vi "Get Pot Zero.vi"() -> (2 "Left Pot 0":dbl, 3 "Right Pot 0":dbl)   [LabVIEW 2015]
uses:
  Common Code/Dashboard Communication/Dashboard Control Data.ctl
  Common Code/Shooter Presets.ctl
  Common Code/Shot Presets.ctl
  Common Code/Encoder Control.ctl
  Common Code/Drivetrain Settings.ctl
  Common Code/Goal Vision Packet.ctl
  Common Code/Dashboard Drivetrain Command.ctl
  Common Code/Drivetrain Vision.ctl
  Common Code/Intake Command Cluster.ctl
  Common Code/Ball Tracking Command Cluster.ctl
  Common Code/Ball Vision Packet.ctl
  Common Code/Tracking Mode.ctl
  Robot Global Data.vi
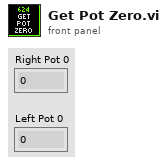
[diagram p1: front panel]
types:
  T1 = typedef "Dashboard Control Data.ctl" = cluster{"Shooter Presets":T2, "Encoder Control":T4, "Steer PID output":cluster{"output high":dbl, "output low":dbl}, " Steer PID gains":cluster{"proportional gain (Kc)":dbl, "integral time (Ti, min)":dbl, "derivative time (Td, min)":dbl}, "Drivetrain Settings":T5, "Vision Packet":T6, "Dashboard Drivetrain Command":T7, "Intake Command Cluster":T9, "Info/Command Cluster":T10, "Ball Vision Packet":T11}
  T2 = typedef "Shooter Presets.ctl" = cluster{"Batter Shot":T3, "Low Bar Curve Shot":T3, "Deep Middle Shot":T3, "Manual Shot":T3, "Left Ticks Per Rotation":dbl, "Right Ticks Per Rotation":dbl, "Low Bar Shot":T3, "Shooter RPM Tolerance":dbl, "IIR Filter Power":dbl, "Trigger Power":dbl, "Fire from Load Delay":i32, "Angle Pot Scale Factor":dbl, "Angle Pot Zero":dbl, "Shooter Deck Length":dbl, "String Pot Dist From Pivot":dbl, "Angle PID gains":cluster{"proportional gain (Kc)":dbl, "integral time (Ti, min)":dbl, "derivative time (Td, min)":dbl}, "Angle Motor Output Range":cluster{"output high":dbl, "output low":dbl}, "Shooter Angle Tolerance":dbl, "Vision Shoot m":dbl, "Vision Shoot b":dbl, "Dist from Axis Cam to Pivot":dbl, "High Goal Center Height":dbl}
  T3 = typedef "Shot Presets.ctl" = cluster{"Left Wheel RPM":dbl, "Right Wheel RPM":dbl, "Angle":dbl}
  T4 = typedef "Encoder Control.ctl" = cluster{"Right Tick Constant":dbl, "Left Tick Constant":dbl, "Reset?":bool, "Y Dist":cluster{"PID gains":cluster{"proportional gain (Kc)":dbl, "integral time (Ti, min)":dbl, "derivative time (Td, min)":dbl}}, "Y Stop Thresh":dbl, "Y Stop Speed":dbl}
  T5 = typedef "Drivetrain Settings.ctl" = cluster{"Gyro Tolerance":dbl, "Throttle Ramp (ms)":dbl, "Angular rate compensation":bool, "Throttle to Rate Scale":dbl, "Rate compensation gain":dbl}
  T6 = typedef "Goal Vision Packet.ctl" = cluster{"Distance":dbl, "Center X":dbl, "Center Y":dbl, "Found Target?":bool}
  T7 = typedef "Dashboard Drivetrain Command.ctl" = cluster{"Drivetrain Vision":T8, "Vision Scale Down Speed":dbl, "Vision PID gains":cluster{"proportional gain (Kc)":dbl, "integral time (Ti, min)":dbl, "derivative time (Td, min)":dbl}}
  T8 = typedef "Drivetrain Vision.ctl" = cluster{"High parameters":dbl, "Low parameters":dbl}
  T9 = typedef "Intake Command Cluster.ctl" = cluster{"Suck Speed":dbl, "Spit Speed":dbl, "Right Pot 0":dbl, "Left Pot 0":dbl, "Trigger Power":dbl, "Raise Speed":dbl, "Lower Speed":dbl}
  T10 = typedef "Ball Tracking Command Cluster.ctl" = cluster{"Distance to Ball":dbl, "Desired Angle":dbl, "Command":enum16{"Turn to Ball", "Turn to Angle", "Get Distance"}, "Pixels from Center":dbl}
  T11 = typedef "Ball Vision Packet.ctl" = cluster{"Ball Detected?":bool, "Distance to Ball":dbl, "Desired Angle":dbl, "Pixels from Center":dbl, "Tracking mode":T12}
  T12 = typedef "Tracking Mode.ctl" = enum16{"Turn to Ball", "Turn to Angle"}
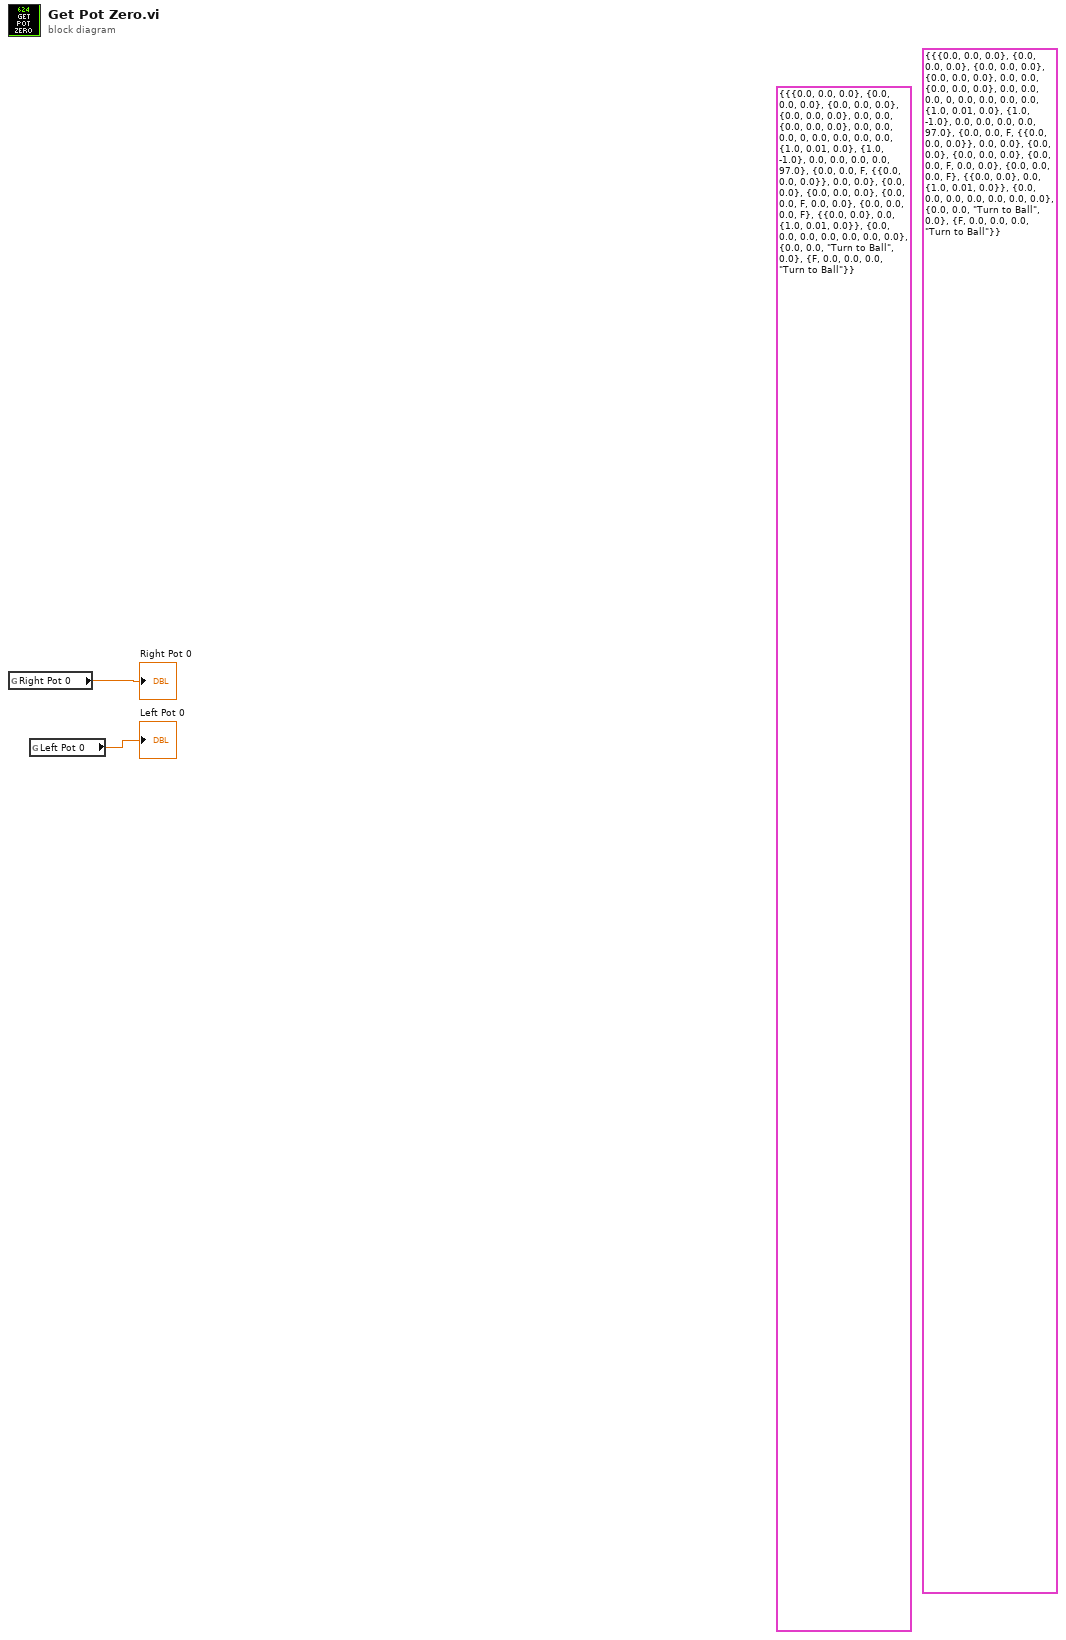
[diagram p0: block diagram]
diagram:
  (unwired) T1 {"Shooter Presets"={"Batter Shot"={"Left Wheel RPM"=0.0, "Right Wheel RPM"=0.0, "Angle"=0.0}, "Low Bar Curve Shot"={"Left Wheel RPM"=0.0, "Right Wheel RPM"=0.0, "Angle"=0.0}, "Deep Middle Shot"={"Left Wheel RPM"=0.0, "Right Wheel RPM"=0.0, "Angle"=0.0}, "Manual Shot"={"Left Wheel RPM"=0.0, "Right Wheel RPM"=0.0, "Angle"=0.0}, "Left Ticks Per Rotation"=0.0, "Right Ticks Per Rotation"=0.0, "Low Bar Shot"={"Left Wheel RPM"=0.0, "Right Wheel RPM"=0.0, "Angle"=0.0}, "Shooter RPM Tolerance"=0.0, "IIR Filter Power"=0.0, "Trigger Power"=0.0, "Fire from Load Delay"=0, "Angle Pot Scale Factor"=0.0, "Angle Pot Zero"=0.0, "Shooter Deck Length"=0.0, "String Pot Dist From Pivot"=0.0, "Angle PID gains"={"proportional gain (Kc)"=1.0, "integral time (Ti, min)"=0.01, "derivative time (Td, min)"=0.0}, "Angle Motor Output Range"={"output high"=1.0, "output low"=-1.0}, "Shooter Angle Tolerance"=0.0, "Vision Shoot m"=0.0, "Vision Shoot b"=0.0, "Dist from Axis Cam to Pivot"=0.0, "High Goal Center Height"=97.0}, "Encoder Control"={"Right Tick Constant"=0.0, "Left Tick Constant"=0.0, "Reset?"=FALSE, "Y Dist"={"PID gains"={"proportional gain (Kc)"=0.0, "integral time (Ti, min)"=0.0, "derivative time (Td, min)"=0.0}}, "Y Stop Thresh"=0.0, "Y Stop Speed"=0.0}, "Steer PID output"={"output high"=0.0, "output low"=0.0}, " Steer PID gains"={"proportional gain (Kc)"=0.0, "integral time (Ti, min)"=0.0, "derivative time (Td, min)"=0.0}, "Drivetrain Settings"={"Gyro Tolerance"=0.0, "Throttle Ramp (ms)"=0.0, "Angular rate compensation"=FALSE, "Throttle to Rate Scale"=0.0, "Rate compensation gain"=0.0}, "Vision Packet"={"Distance"=0.0, "Center X"=0.0, "Center Y"=0.0, "Found Target?"=FALSE}, "Dashboard Drivetrain Command"={"Drivetrain Vision"={"High parameters"=0.0, "Low parameters"=0.0}, "Vision Scale Down Speed"=0.0, "Vision PID gains"={"proportional gain (Kc)"=1.0, "integral time (Ti, min)"=0.01, "derivative time (Td, min)"=0.0}}, "Intake Command Cluster"={"Suck Speed"=0.0, "Spit Speed"=0.0, "Right Pot 0"=0.0, "Left Pot 0"=0.0, "Trigger Power"=0.0, "Raise Speed"=0.0, "Lower Speed"=0.0}, "Info/Command Cluster"={"Distance to Ball"=0.0, "Desired Angle"=0.0, "Command"=enum."Turn to Ball", "Pixels from Center"=0.0}, "Ball Vision Packet"={"Ball Detected?"=FALSE, "Distance to Ball"=0.0, "Desired Angle"=0.0, "Pixels from Center"=0.0, "Tracking mode"=enum."Turn to Ball"}} ("Dashboard Control Data")
  (unwired) T1 {"Shooter Presets"={"Batter Shot"={"Left Wheel RPM"=0.0, "Right Wheel RPM"=0.0, "Angle"=0.0}, "Low Bar Curve Shot"={"Left Wheel RPM"=0.0, "Right Wheel RPM"=0.0, "Angle"=0.0}, "Deep Middle Shot"={"Left Wheel RPM"=0.0, "Right Wheel RPM"=0.0, "Angle"=0.0}, "Manual Shot"={"Left Wheel RPM"=0.0, "Right Wheel RPM"=0.0, "Angle"=0.0}, "Left Ticks Per Rotation"=0.0, "Right Ticks Per Rotation"=0.0, "Low Bar Shot"={"Left Wheel RPM"=0.0, "Right Wheel RPM"=0.0, "Angle"=0.0}, "Shooter RPM Tolerance"=0.0, "IIR Filter Power"=0.0, "Trigger Power"=0.0, "Fire from Load Delay"=0, "Angle Pot Scale Factor"=0.0, "Angle Pot Zero"=0.0, "Shooter Deck Length"=0.0, "String Pot Dist From Pivot"=0.0, "Angle PID gains"={"proportional gain (Kc)"=1.0, "integral time (Ti, min)"=0.01, "derivative time (Td, min)"=0.0}, "Angle Motor Output Range"={"output high"=1.0, "output low"=-1.0}, "Shooter Angle Tolerance"=0.0, "Vision Shoot m"=0.0, "Vision Shoot b"=0.0, "Dist from Axis Cam to Pivot"=0.0, "High Goal Center Height"=97.0}, "Encoder Control"={"Right Tick Constant"=0.0, "Left Tick Constant"=0.0, "Reset?"=FALSE, "Y Dist"={"PID gains"={"proportional gain (Kc)"=0.0, "integral time (Ti, min)"=0.0, "derivative time (Td, min)"=0.0}}, "Y Stop Thresh"=0.0, "Y Stop Speed"=0.0}, "Steer PID output"={"output high"=0.0, "output low"=0.0}, " Steer PID gains"={"proportional gain (Kc)"=0.0, "integral time (Ti, min)"=0.0, "derivative time (Td, min)"=0.0}, "Drivetrain Settings"={"Gyro Tolerance"=0.0, "Throttle Ramp (ms)"=0.0, "Angular rate compensation"=FALSE, "Throttle to Rate Scale"=0.0, "Rate compensation gain"=0.0}, "Vision Packet"={"Distance"=0.0, "Center X"=0.0, "Center Y"=0.0, "Found Target?"=FALSE}, "Dashboard Drivetrain Command"={"Drivetrain Vision"={"High parameters"=0.0, "Low parameters"=0.0}, "Vision Scale Down Speed"=0.0, "Vision PID gains"={"proportional gain (Kc)"=1.0, "integral time (Ti, min)"=0.01, "derivative time (Td, min)"=0.0}}, "Intake Command Cluster"={"Suck Speed"=0.0, "Spit Speed"=0.0, "Right Pot 0"=0.0, "Left Pot 0"=0.0, "Trigger Power"=0.0, "Raise Speed"=0.0, "Lower Speed"=0.0}, "Info/Command Cluster"={"Distance to Ball"=0.0, "Desired Angle"=0.0, "Command"=enum."Turn to Ball", "Pixels from Center"=0.0}, "Ball Vision Packet"={"Ball Detected?"=FALSE, "Distance to Ball"=0.0, "Desired Angle"=0.0, "Pixels from Center"=0.0, "Tracking mode"=enum."Turn to Ball"}} ("Dashboard Control Data")
  n1 = global read "Robot Global Data.vi" "Right Pot 0"() -> (→"Right Pot 0":dbl)
  n2 = global read "Robot Global Data.vi" "Left Pot 0"() -> (→"Left Pot 0":dbl)
